vi "AutoRenameFile.vi"(7 "Contents":string, 8 "error in":errorcluster, 11 "Filename":path) -> (0 "error out":errorcluster)   [LabVIEW 2010]
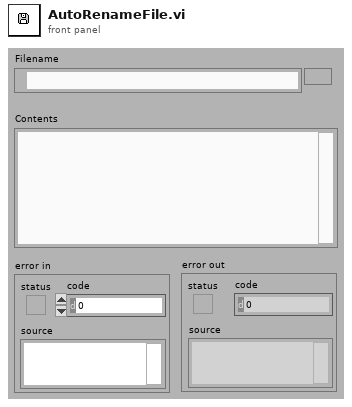
[diagram p1: front panel]
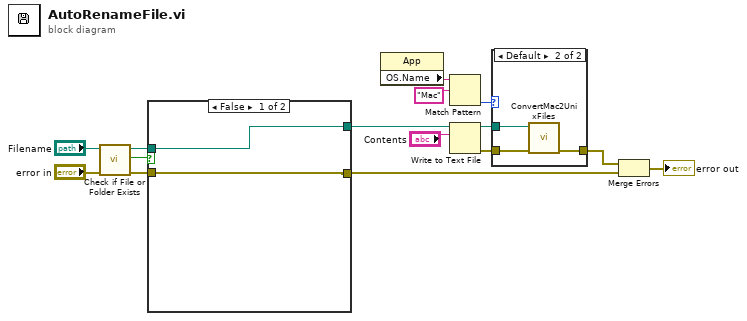
[diagram p0: block diagram]
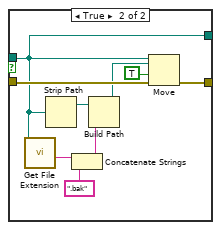
[diagram p3: hidden frame]
diagram:
  n1 = call <vilib>:"Check if File or Folder Exists.vi"("error in (no error)"="error in", "path"="Filename") -> ("error out"=w12:errorcluster, "file or folder exists?"=w13:bool, "dup path"=w10:path)  [unwired: 7 in]
  n2 = case shown="False" w13 {
    tunnel: w12 -> [w16 w25]
    tunnel: w10 -> [w15 w17]
    tunnel: [w15 w17] -> w2
    tunnel: [w16 w18] -> w7
    frame False {
    }
    frame True {
      n3 = call <vilib>:"Get File Extension.vi"("file"=w17) -> ("filename without extension"=w23:string)  [unwired: 7 in, 3 out]
      n4 = Strip Path(path=w17) -> (stripped path=w24:path)  [unwired: 1 out]
      n5 = Concatenate Strings(w23, ".bak" ("string")) -> (w21:string)
      n6 = Build Path(base path=w24, name or relative path=w21) -> (appended path=w20:path)
      n7 = Move(source path=w17, error in=w25, 9:TRUE ("overwrite (F)"), 10:w20) -> (error out=w18:errorcluster)  [unwired: 1 in, 2 out]
    }
  }
  n8 = property class="App"() -> ("OS.Name"=w5:string)  [unwired: 2 in, 2 out]
  n9 = Match Pattern(string=w5, regular expression="Mac") -> (offset past match=w4:i32)  [unwired: 1 in, 3 out]
  n10 = Write to Text File(file (use dialog)=w2, text="Contents") -> (error out=w3:errorcluster)  [unwired: 2 in, 2 out]
  n11 = case shown="Default" w4 {
    tunnel: w3 -> [w26 w29]
    tunnel: w2 -> [_ w28]
    tunnel: [w26 w27] -> w1
    frame -1 {
    }
    frame Default {
      n12 = call "ConvertMac2UnixFiles.vi"("Error In"=w29, "Filename"=w28) -> ("Error Out"=w27:errorcluster)  [unwired: 9 in]
    }
  }
  n13 = Merge Errors(w1, w7) -> (→"error out":errorcluster)
